vi "Single Phase Motor Speed Controller.vi"() -> ()   [LabVIEW 2023]
uses:
  <vilib>/Instr/_visa.llb/VISA Configure Serial Port (Instr).vi
  <vilib>/addons/control/pid/pid.llb/PID (DBL).vi
  <vilib>/addons/control/pid/NI_PID_pid.lvlib
panel:
  in  "LabVIEW User Interface":enum32{"Page 1", "Page 2"}(tab)
  in  "Communication Port":refnum<visa-resource-name>
  in  "Stop Software":bool
  in  "Start Button":bool
  in  "Reverse Button":bool
  in  "Stop Button":bool
  in  "Speed Up Button":bool
  in  "Slow Down Button":bool
  out "Voltage, V":dbl format="%#1_3f"
  out "Current, A":dbl format="%#1_3f"
  out "Power, W":dbl format="%#1_3f"
  out "Current Speed, RPM":dbl
  in  "Forward Button":bool
  out "Status":string
  out "Speed Gauge":dbl(knob) scale=0.0..5000.0
  out "Voltmeter, V":dbl(knob) scale=45.0..75.0
  out "Ammeter, A":dbl(knob) scale=0.0..1.5
  in  "Set RPM Speed":dbl=3500.0 min=800.0 max=3500.0
  in  "PID Speed Controller":bool
  out "PID Gains":T1={"Proportional"=1.0, "Integral"=0.01, "Derivative"=0.0} {"Derivative" format="%.4f"; "Integral" format="%.3f"; "Proportional" format="%.3f"}
  out "PID Signal":dbl format="%#_2g"
  out "Steady State Error":dbl
  out "Speed Response Chart":cluster{"Set RPM Speed":dbl, dbl}(graph)
  out "Setpoint Speed":dbl
  out "Actual Speed":dbl
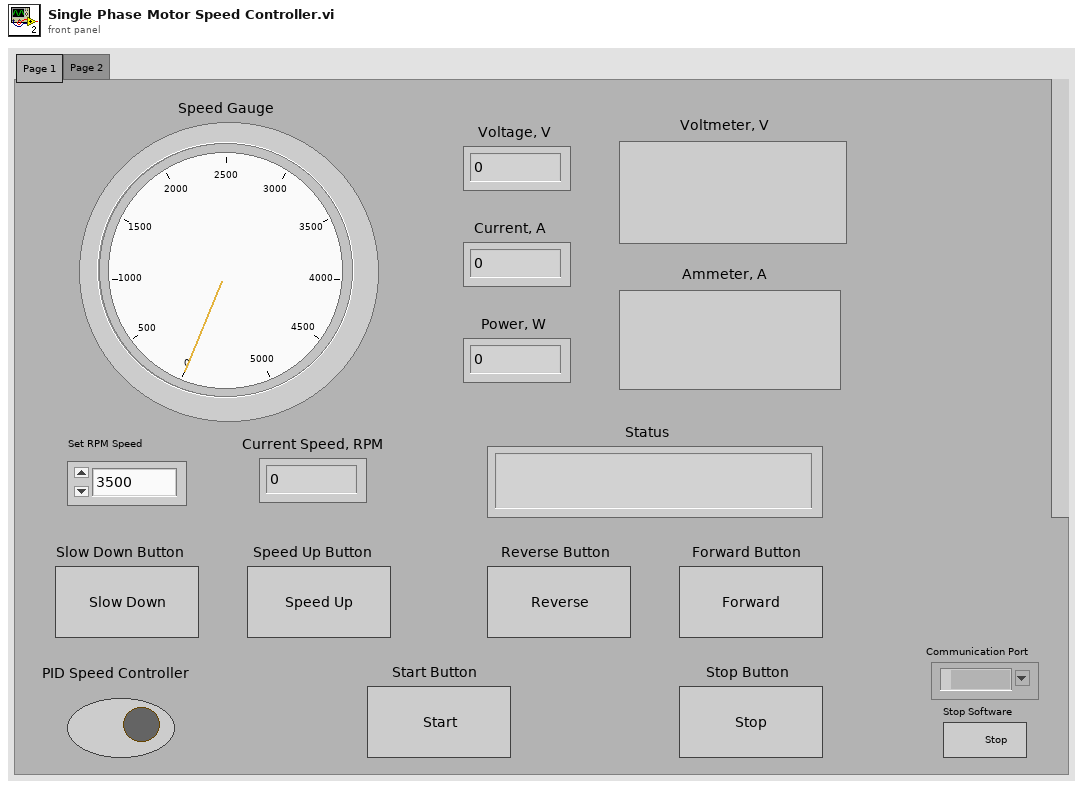
[diagram p1: front panel]
types:
  T1 = cluster{"Proportional":dbl, "Integral":dbl, "Derivative":dbl}
  T2 = cluster{"proportional gain (Kc)":dbl, "integral time (Ti, min)":dbl, "derivative time (Td, min)":dbl}
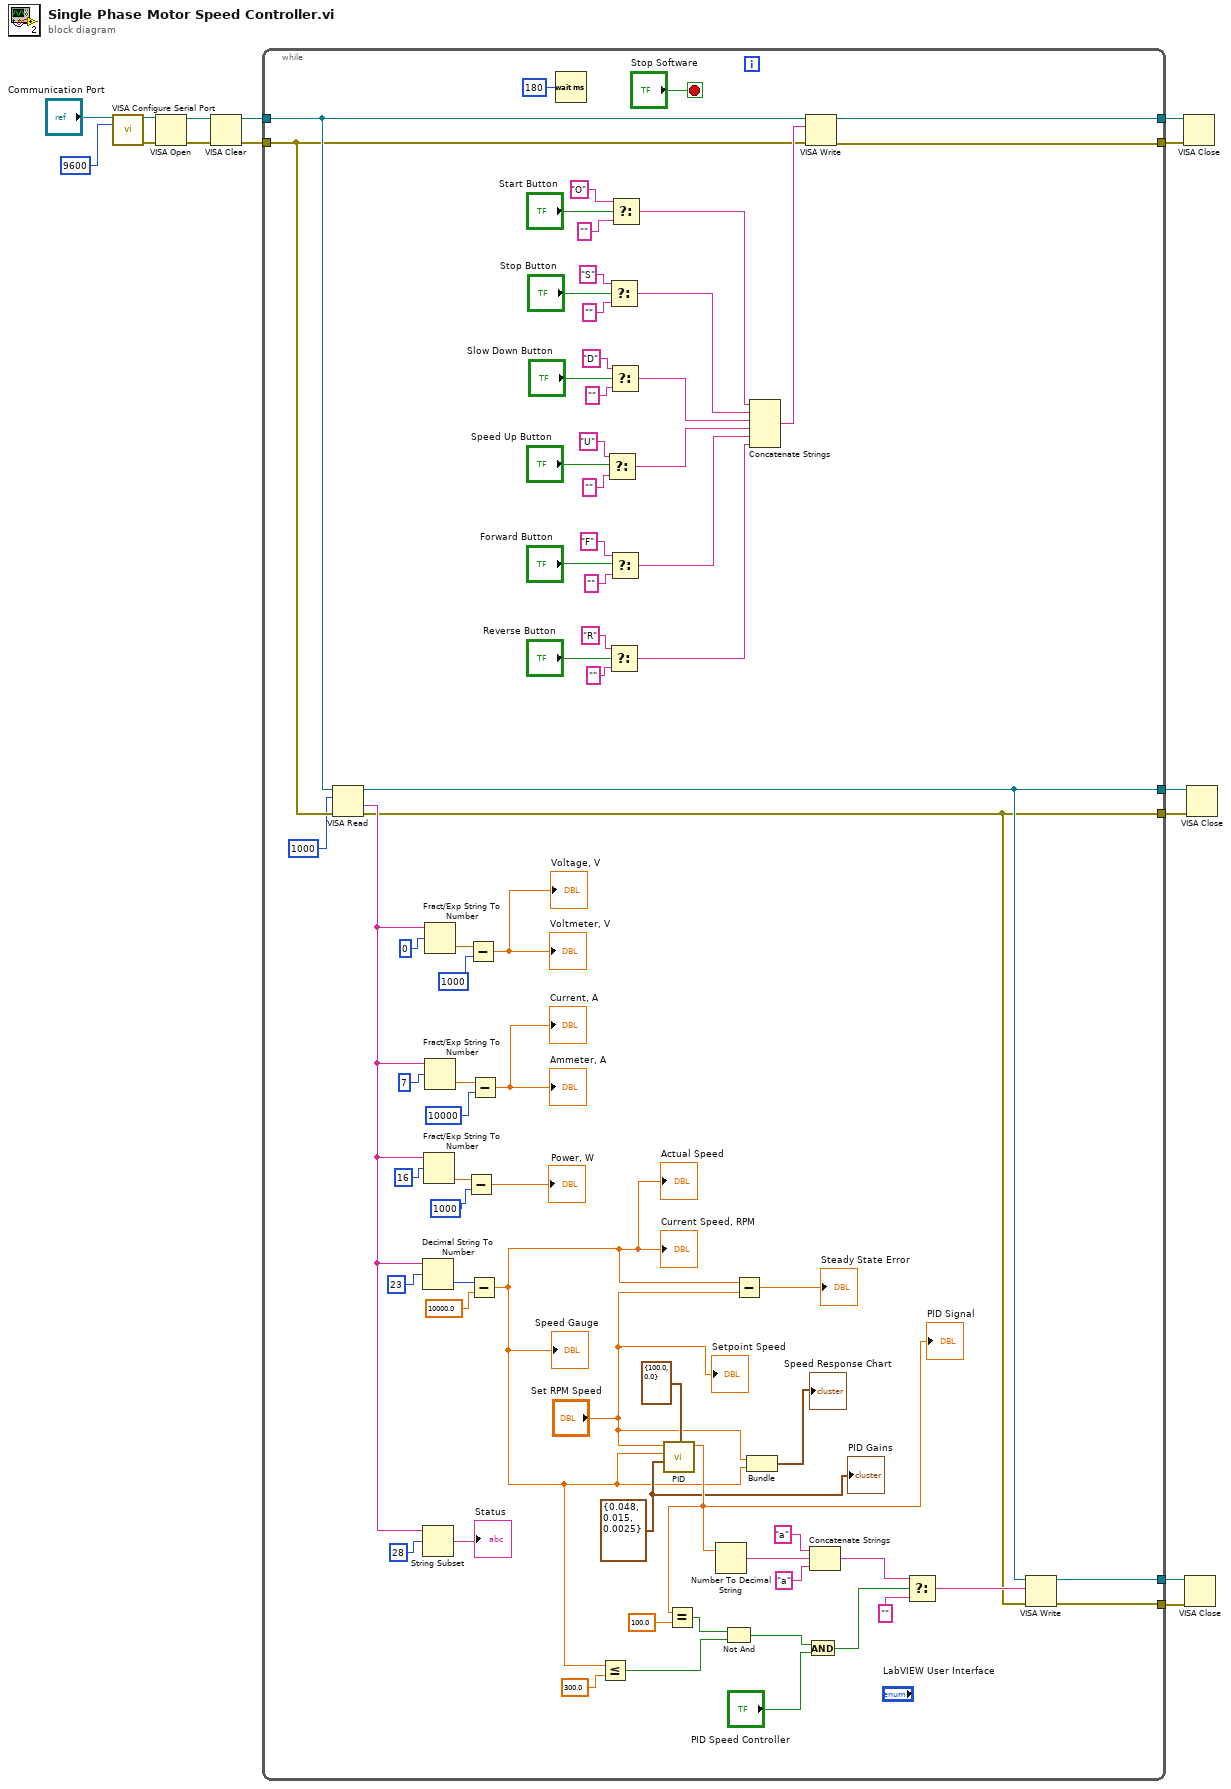
[diagram p0: block diagram]
diagram:
  n1 = call-poly "VISA Configure Serial Port"("VISA resource name"="Communication Port", "baud rate (9600)"=u32 9600) -> ("VISA resource name out"=w12:refnum<visa-resource-name>, "error out"=w11:errorcluster)  [unwired: 12 in]
  n2 = VISA Open(error in (no error)=w11, VISA resource name=w12) -> (VISA resource name=w2:refnum<visa-resource-name>, error out=w1:errorcluster)  [unwired: 3 in]
  n3 = VISA Clear(VISA resource name=w2, error in (no error)=w1) -> (VISA resource name out=w4:refnum<visa-resource-name>, error out=w3:errorcluster)
  n4 = while {
    tunnel: [w61] -> w8
    tunnel: w4 -> [w40]
    tunnel: w3 -> [w39]
    tunnel: [w60] -> w9
    tunnel: [w34] -> w7
    tunnel: [w29] -> w10
    tunnel: [w31] -> w6
    tunnel: [w30] -> w5
    stop <- "Stop Software" stop-if-true
    w17 = T2 {"proportional gain (Kc)"=0.048, "integral time (Ti, min)"=0.015, "derivative time (Td, min)"=0.0025} ("PID gains")
    n5 = VISA Read(VISA resource name=w40, byte count=u32 1000, error in (no error)=w39) -> (VISA resource name out=w34:refnum<visa-resource-name>, read buffer=w36:string, error out=w31:errorcluster)  [unwired: 1 out]
    n6 = Decimal String To Number(string=w36, offset=23) -> (number=w43:i32)  [unwired: 1 in, 1 out]
    n7 = String Subset(string=w36, offset (0)=28) -> (substring=→"Status":string)  [unwired: 1 in]
    n8 = Fract/Exp String To Number(string=w36, offset=16) -> (number=w49:dbl)  [unwired: 2 in, 1 out]
    n9 = Fract/Exp String To Number(string=w36, offset=0) -> (number=w51:dbl)  [unwired: 2 in, 1 out]
    n10 = Fract/Exp String To Number(string=w36, offset=7) -> (number=w50:dbl)  [unwired: 2 in, 1 out]
    n11 = Subtract(x=w49, y=1000) -> (x-y=→"Power, W":dbl)
    n12 = Subtract(x=w51, y=1000) -> (x-y=→"Voltage, V" →"Voltmeter, V":dbl)
    n13 = Subtract(x=w43, y=10000.0) -> (x-y=w16:dbl)
    "Current Speed, RPM" <- w16
    "Speed Gauge" <- w16
    "Actual Speed" <- w16
    n14 = Subtract(x=w50, y=10000) -> (x-y=→"Current, A" →"Ammeter, A":dbl)
    n15 = Wait (ms)(milliseconds to wait=u32 180) -> ()  [unwired: 1 out]
    n16 = Less Or Equal?(x=w16, y=300.0) -> (x <= y?=w23:bool)
    n17 = Select(t="U", s="Speed Up Button", f="") -> (s? t:f=w85:string)
    n18 = Select(t="S", s="Stop Button", f="") -> (s? t:f=w83:string)
    n19 = Select(t="R", s="Reverse Button", f="") -> (s? t:f=w87:string)
    n20 = Select(t="D", s="Slow Down Button", f="") -> (s? t:f=w84:string)
    n21 = Select(t="F", s="Forward Button", f="") -> (s? t:f=w86:string)
    n22 = Select(t="O", s="Start Button", f="") -> (s? t:f=w82:string)
    n23 = call-poly <vilib>:"PID.vi"("output range"=cluster{"output high":dbl, "output low":dbl} {"output high"=100.0, "output low"=0.0}, "PID gains"=w17, "process variable"=w16, "setpoint"="Set RPM Speed") -> ("output"=w18:dbl)  [unwired: 6 in, 1 out]
    "PID Signal" <- w18
    n24 = Equal?(x=w18, y=100.0) -> (x = y?=w24:bool)
    n25 = Number To Decimal String(number=w18) -> (decimal integer string=w62:string)  [unwired: 1 in]
    n26 = Not And(1:w23, 2:w24) -> (0:w22:bool)
    n27 = Subtract(x=w16, y="Set RPM Speed") -> (x-y=→"Steady State Error":dbl)
    n28 = Bundle("Set RPM Speed"="Set RPM Speed", w16) -> (→"Speed Response Chart":cluster{"Set RPM Speed":dbl, dbl})  [unwired: 1 in]
    n29 = Concatenate Strings(w82, w83, w84, w85, w86, w87) -> (w64:string)
    n30 = VISA Write(VISA resource name=w40, write buffer=w64, error in (no error)=w39) -> (VISA resource name out=w60:refnum<visa-resource-name>, error out=w61:errorcluster)  [unwired: 1 out]
    n31 = And(x=w22, y="PID Speed Controller") -> (x .and. y?=w28:bool)
    n32 = Concatenate Strings("a" ("string"), w62, "a" ("string")) -> (w56:string)
    n33 = Select(t=w56, s=w28, f="") -> (s? t:f=w37:string)
    n34 = VISA Write(VISA resource name=w34, write buffer=w37, error in (no error)=w31) -> (VISA resource name out=w30:refnum<visa-resource-name>, error out=w29:errorcluster)  [unwired: 1 out]
    "PID Gains" <- w17
    "Setpoint Speed" <- "Set RPM Speed"
  }
  n35 = VISA Close(VISA resource name=w9, error in (no error)=w8) -> ()  [unwired: 1 out]
  n36 = VISA Close(VISA resource name=w5, error in (no error)=w10) -> ()  [unwired: 1 out]
  n37 = VISA Close(VISA resource name=w7, error in (no error)=w6) -> ()  [unwired: 1 out]
